vi "ReDraw ROI.vi"(6 "Mode (Redraw All)":T1, 8 "error in":errorcluster, 10 "Selected/Deselected":i32[](array[numeric]), 11 "XYZ Coordinates":T2[](array[typedef]) {"Apparent Frame Size" format="%#_6f"; "Original FOV (um)" format="%#_6f"; "Pixels per miniscan" format="%#_6f"; "Dwell Time per pixel" format="%#_6f"; "Resolution" format="%#_6f"; "ROI group ID" format="%#_6f"; "Laser Power (%)" format="%#_6f"; "Zoom" format="%#_6f"; "Frame Size" format="%#_6f"; "Number of lines" format="%#_6f"; "Composite ID" format="%#_6f"; "Angle (deg)" format="%#_6f"; "ROI Time (ns)" format="%#_6f"; "ROI ID" format="%#_6f"; "Pixels in ROI" format="%#_6f"; "ROI index" format="%#_6f"; "Z stop" format="%#_6f"; "Y stop" format="%#_6f"; "X stop" format="%#_6f"; "Z start" format="%#_6f"; "X start" format="%#_6f"; "Y start" format="%#_6f"}) -> (0 "error out":errorcluster)   [LabVIEW 2020]
uses:
  Visualisation/Functional Imaging Viewer/Typedefs/ROI parameters data type.ctl
  Typedefs/Redraw ROI.ctl
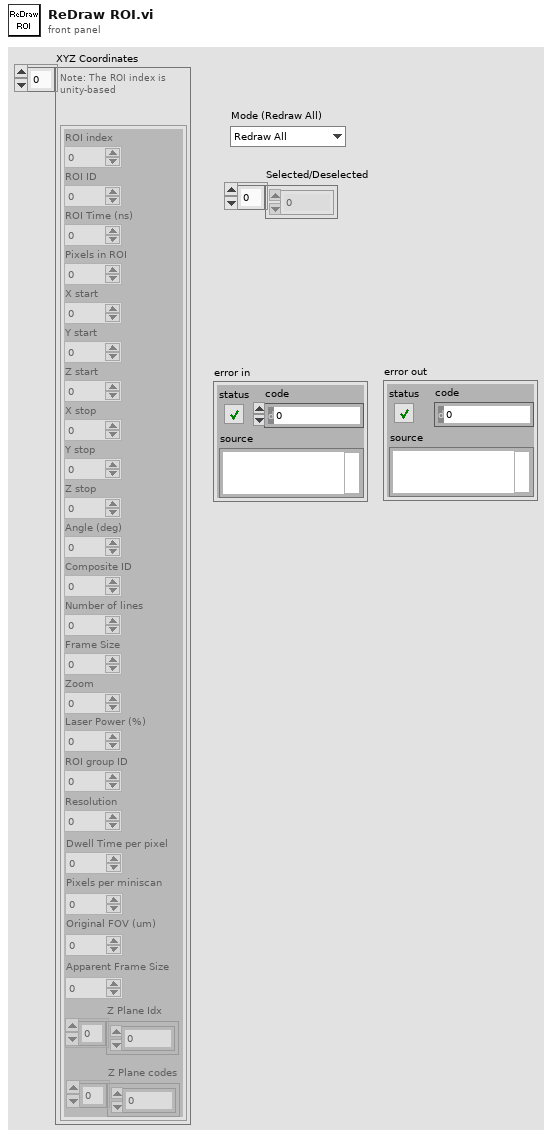
[diagram p1: front panel]
types:
  T1 = typedef "Redraw ROI.ctl" = enum16{"Redraw All", "Redraw Deselected", "Draw Last", "Redraw Selected"}
  T2 = typedef "ROI parameters data type.ctl" = cluster{"ROI index":dbl, "ROI ID":dbl, "ROI Time (ns)":dbl, "Pixels in ROI":dbl, "X start":dbl, "Y start":dbl, "Z start":dbl, "X stop":dbl, "Y stop":dbl, "Z stop":dbl, "Angle (deg)":dbl, "Composite ID":dbl, "Number of lines":dbl, "Frame Size":dbl, "Zoom":dbl, "Laser Power (%)":dbl, "ROI group ID":dbl, "Resolution":dbl, "Dwell Time per pixel":dbl, "Pixels per miniscan":dbl, "Original FOV (um)":dbl, "Apparent Frame Size":dbl, "Z Plane Idx":i32[], "Z Plane codes":i32[]}
  T3 = typedef "IMAQ Image.ctl" = refnum<image>
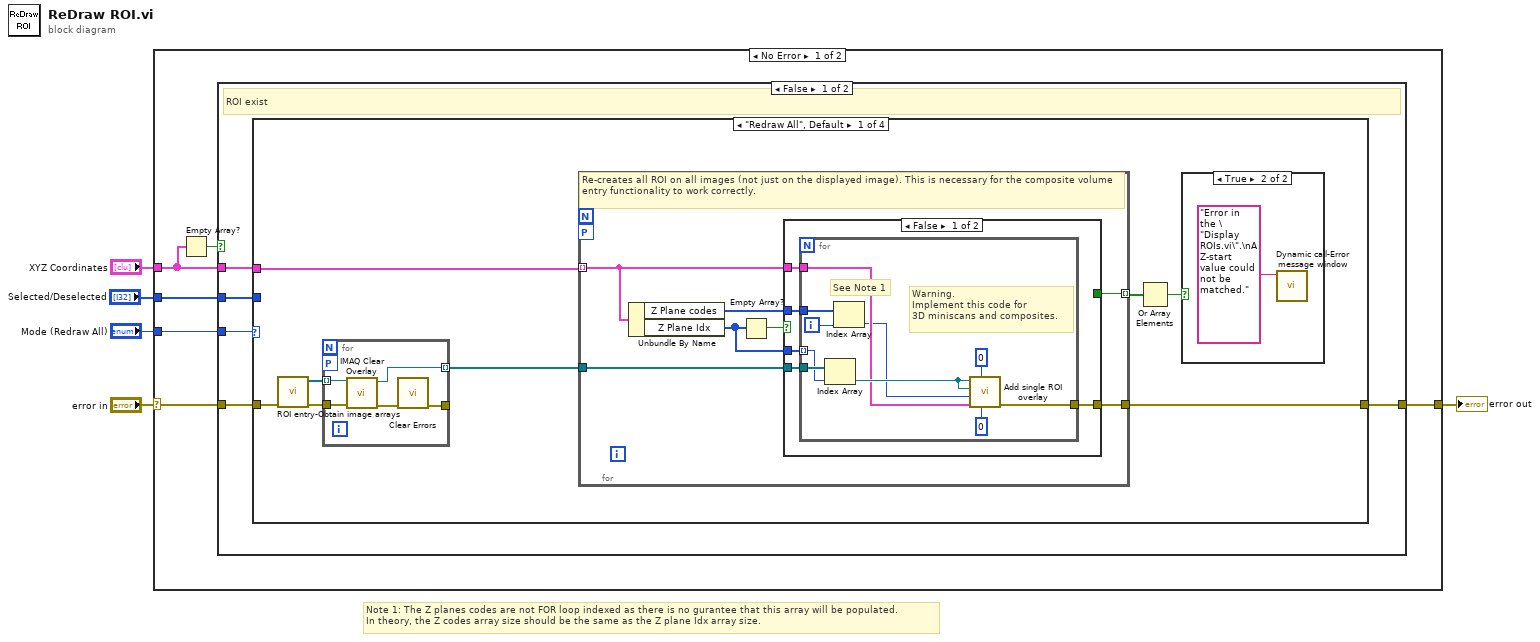
[diagram p0: block diagram]
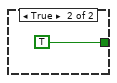
[diagram p3: hidden frame]
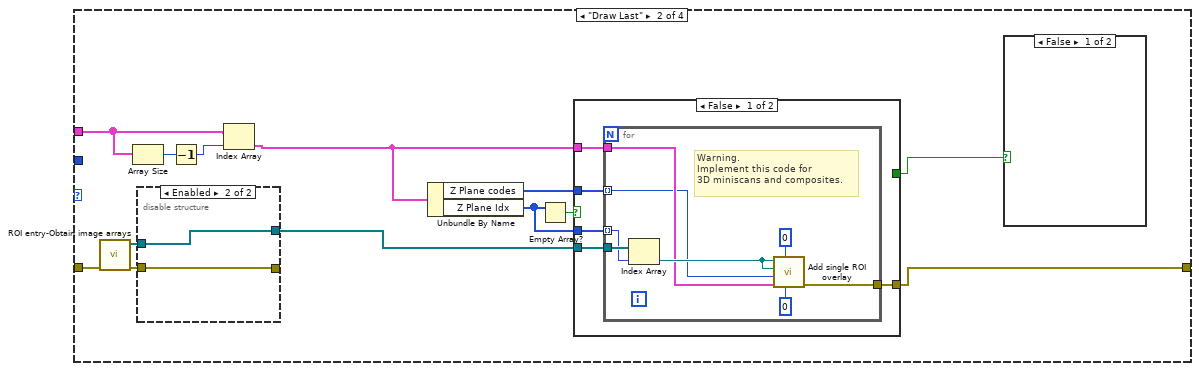
[diagram p4: hidden frame]
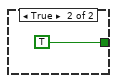
[diagram p5: hidden frame]
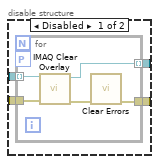
[diagram p6: hidden frame]
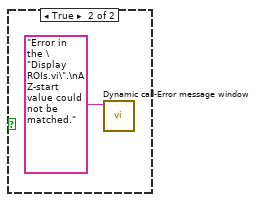
[diagram p7: hidden frame]
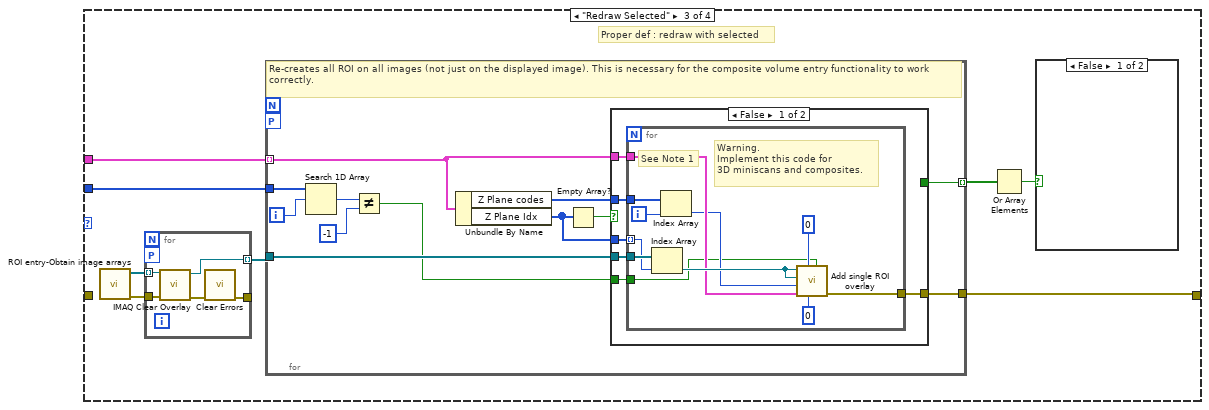
[diagram p8: hidden frame]
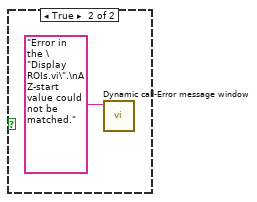
[diagram p9: hidden frame]
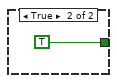
[diagram p10: hidden frame]
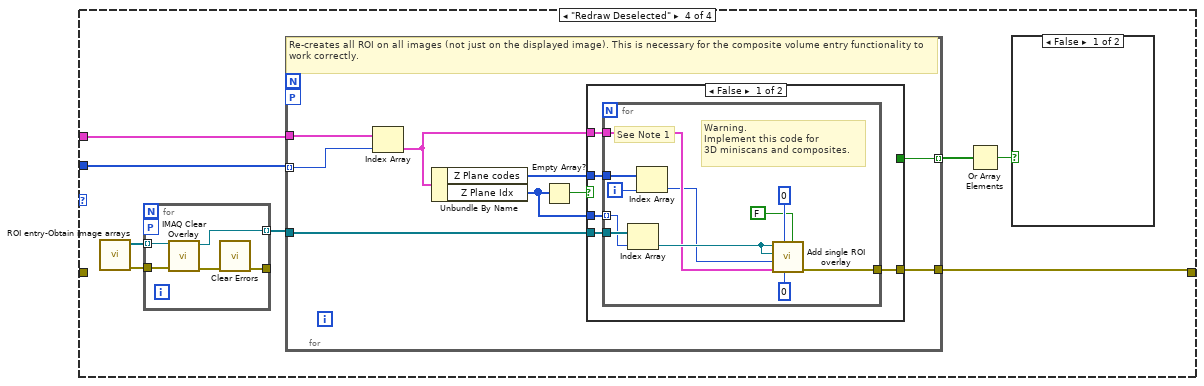
[diagram p11: hidden frame]
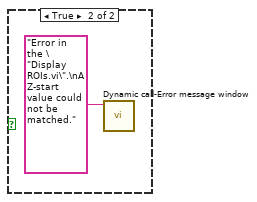
[diagram p12: hidden frame]
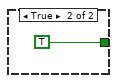
[diagram p13: hidden frame]
diagram:
  # "Note 1: The Z planes codes are not FOR loop indexed as there is no gurantee that this array will be populated.\nIn theory, the Z codes array size should be the same as the Z plane Idx array size."
  n1 = case shown="No Error" "error in" {
    selector: "error in" -> [w9 w178]
    tunnel: "XYZ Coordinates" -> [w11 _]
    tunnel: [w10 w178] -> w3
    tunnel: "Mode (Redraw All)" -> [w7 _]
    tunnel: "Selected/Deselected" -> [w6 _]
    frame No Error {
      n2 = Empty Array?(array=w11) -> (empty?=w8:bool)
      n3 = case shown="False" w8 {
        tunnel: w11 -> [w16 _]
        tunnel: [w15 w177] -> w10
        tunnel: w9 -> [w14 w177]
        tunnel: w7 -> [w13 _]
        tunnel: w6 -> [w12 _]
        frame False {
          # "ROI exist"
          n4 = case shown="\"Redraw All\", Default" w13 {
            tunnel: w16 -> [w24 w56 w94 w139]
            tunnel: [w20 w58 w95 w137] -> w15
            tunnel: w14 -> [w17 w64 _ _]
            tunnel: w12 -> [_ _ w93 w138]
            frame "Redraw All", Default {
              n5 = call "ROI entry-Obtain image arrays.vi"("error in (no error)"=w17) -> ("error IO"=w18:errorcluster, "RedImageArray"=w19:T3[])  [unwired: 9 in]
              n6 = for {
                tunnel: w19 -> [w30] mode=indexing
                tunnel: [w29] -> w23 mode=indexing
                workers-P: _ -> [_]
                tunnel: [w27] -> _
                tunnel: w18 -> [w26]
                n7 = call "IMAQ Clear Overlay"("error in (no error)"=w26, "Image"=w30) -> ("error out"=w28:errorcluster, "Image Out"=w29:T3)  [unwired: 8 in]
                n8 = call <vilib>:"Clear Errors.vi"("error in (no error)"=w28) -> ("error out"=w27:errorcluster)  [unwired: 5 in, 1 out]
              }
              n9 = for {
                tunnel: w24 -> [w33] mode=indexing
                tunnel: w23 -> [w37]
                workers-P: _ -> [_]
                tunnel: [w36] -> w22 mode=indexing
                tunnel: [w35] -> w20
                # "Re-creates all ROI on all images (not just on the displayed image). This is necessary for the composite volume entry functionality to work correctly."
                n10 = Unbundle By Name(w33) -> ("Z Plane codes"=w32:i32[], "Z Plane Idx"=w31:i32[])
                n11 = Empty Array?(array=w31) -> (empty?=w34:bool)
                n12 = case shown="False" w34 {
                  tunnel: w37 -> [w42 _]
                  tunnel: w33 -> [w41 _]
                  tunnel: [_ TRUE] -> w36
                  tunnel: [w40 _] -> w35
                  tunnel: w32 -> [w38 _]
                  tunnel: w31 -> [w39 _]
                  frame False {
                    n13 = for {
                      tunnel: w42 -> [w52]
                      tunnel: w41 -> [w50]
                      tunnel: [w47] -> w40
                      tunnel: w39 -> [w46] mode=indexing
                      tunnel: w38 -> [w45]
                      i -> [w44]
                      # "See Note 1"
                      # "Warning.\nImplement this code for\n3D miniscans and composites."
                      n14 = Index Array(array=w52, index=w46) -> (element=w51:T3)
                      n15 = Index Array(array=w45, index=w44) -> (element=w43:i32)
                      n16 = call "Add single ROI overlay.vi"("Abs. index of selected Z-plane (unity-based)"=0, "Number of Z-planes"=0, "ROI Properties"=w50, "Z code"=w43, "Image2"=w51, "Image1"=w51) -> ("Error out"=w47:errorcluster)  [unwired: 3 in, 2 out]
                    }
                  }
                  frame True {
                  }
                }
              }
              n17 = Or Array Elements(Boolean array=w22) -> (logical OR=w21:bool)
              n18 = case shown="True" w21 {
                frame False {
                }
                frame True {
                  n19 = call "Dynamic call-Error message window.vi"("Error Message"="Error in the \"Display ROIs.vi\".\nA Z-start value could not be matched.") -> ()  [unwired: 10 in, 1 out]
                }
              }
            }
            frame "Draw Last" {
              n20 = call "ROI entry-Obtain image arrays.vi"("error in (no error)"=w64) -> ("error IO"=w65:errorcluster, "RedImageArray"=w66:T3[])  [unwired: 9 in]
              n21 = Array Size(array=w56) -> (size(s)=w55:i32)
              n22 = disable-structure shown="Enabled" {
                disable-tunnel: [w84 w91] -> w60
                disable-tunnel: [w83 w90] -> _
                disable-tunnel: w66 -> [w82 w91]
                disable-tunnel: w65 -> [w81 w90]
                frame Disabled {
                  n23 = for {
                    tunnel: w82 -> [w89] mode=indexing
                    tunnel: [w88] -> w84 mode=indexing
                    workers-P: _ -> [_]
                    tunnel: [w86] -> w83
                    tunnel: w81 -> [w85]
                    n24 = call "IMAQ Clear Overlay"("error in (no error)"=w85, "Image"=w89) -> ("error out"=w87:errorcluster, "Image Out"=w88:T3)  [unwired: 8 in]
                    n25 = call <vilib>:"Clear Errors.vi"("error in (no error)"=w87) -> ("error out"=w86:errorcluster)  [unwired: 5 in, 1 out]
                  }
                }
                frame Enabled {
                }
              }
              n26 = Decrement(x=w55) -> (x-1=w54:i32)
              n27 = Index Array(array=w56, index=w54) -> (element=w57:T2)
              n28 = Unbundle By Name(w57) -> ("Z Plane codes"=w62:i32[], "Z Plane Idx"=w61:i32[])
              n29 = Empty Array?(array=w61) -> (empty?=w63:bool)
              n30 = case shown="False" w63 {
                tunnel: w60 -> [w71 _]
                tunnel: w57 -> [w70 _]
                tunnel: [_ TRUE] -> w59
                tunnel: [w69 _] -> w58
                tunnel: w62 -> [w67 _]
                tunnel: w61 -> [w68 _]
                frame False {
                  n31 = for {
                    tunnel: w71 -> [w79]
                    tunnel: w70 -> [w77]
                    tunnel: [w74] -> w69
                    tunnel: w68 -> [w73] mode=indexing
                    tunnel: w67 -> [w72] mode=indexing
                    # "Warning.\nImplement this code for\n3D miniscans and composites."
                    n32 = Index Array(array=w79, index=w73) -> (element=w78:T3)
                    n33 = call "Add single ROI overlay.vi"("Abs. index of selected Z-plane (unity-based)"=0, "Number of Z-planes"=0, "ROI Properties"=w77, "Z code"=w72, "Image2"=w78, "Image1"=w78) -> ("Error out"=w74:errorcluster)  [unwired: 3 in, 2 out]
                  }
                }
                frame True {
                }
              }
              n34 = case shown="False" w59 {
                frame False {
                }
                frame True {
                  n35 = call "Dynamic call-Error message window.vi"("Error Message"="Error in the \"Display ROIs.vi\".\nA Z-start value could not be matched.") -> ()  [unwired: 10 in, 1 out]
                }
              }
            }
            frame "Redraw Selected" {
              # "Proper def : redraw with selected"
              n36 = call "ROI entry-Obtain image arrays.vi"() -> ("error IO"=w99:errorcluster, "RedImageArray"=w100:T3[])  [unwired: 10 in]
              n37 = for {
                tunnel: w100 -> [w136] mode=indexing
                tunnel: [w135] -> w96 mode=indexing
                workers-P: _ -> [_]
                tunnel: [w133] -> _
                tunnel: w99 -> [w132]
                n38 = call "IMAQ Clear Overlay"("error in (no error)"=w132, "Image"=w136) -> ("error out"=w134:errorcluster, "Image Out"=w135:T3)  [unwired: 8 in]
                n39 = call <vilib>:"Clear Errors.vi"("error in (no error)"=w134) -> ("error out"=w133:errorcluster)  [unwired: 5 in, 1 out]
              }
              n40 = for {
                tunnel: w96 -> [w113]
                workers-P: _ -> [_]
                tunnel: [w112] -> w98 mode=indexing
                tunnel: [w111] -> w95
                tunnel: w94 -> [w107] mode=indexing
                tunnel: w93 -> [w106]
                i -> [w105]
                # "Re-creates all ROI on all images (not just on the displayed image). This is necessary for the composite volume entry functionality to work correctly."
                n41 = Search 1D Array(1D array=w106, element=w105) -> (index of element=w104:i32)  [unwired: 1 in]
                n42 = Not Equal?(x=w104, y=-1) -> (x != y?=w102:bool)
                n43 = Unbundle By Name(w107) -> ("Z Plane codes"=w109:i32[], "Z Plane Idx"=w108:i32[])
                n44 = Empty Array?(array=w108) -> (empty?=w110:bool)
                n45 = case shown="False" w110 {
                  tunnel: w113 -> [w119 _]
                  tunnel: w107 -> [w118 _]
                  tunnel: [_ TRUE] -> w112
                  tunnel: [w117 _] -> w111
                  tunnel: w109 -> [w115 _]
                  tunnel: w108 -> [w116 _]
                  tunnel: w102 -> [w114 _]
                  frame False {
                    n46 = for {
                      tunnel: w119 -> [w130]
                      tunnel: w118 -> [w128]
                      tunnel: [w125] -> w117
                      tunnel: w116 -> [w124] mode=indexing
                      tunnel: w115 -> [w123]
                      tunnel: w114 -> [w120]
                      i -> [w122]
                      # "See Note 1"
                      # "Warning.\nImplement this code for\n3D miniscans and composites."
                      n47 = Index Array(array=w130, index=w124) -> (element=w129:T3)
                      n48 = Index Array(array=w123, index=w122) -> (element=w121:i32)
                      n49 = call "Add single ROI overlay.vi"("Selected ?"=w120, "Abs. index of selected Z-plane (unity-based)"=0, "Number of Z-planes"=0, "ROI Properties"=w128, "Z code"=w121, "Image2"=w129, "Image1"=w129) -> ("Error out"=w125:errorcluster)  [unwired: 2 in, 2 out]
                    }
                  }
                  frame True {
                  }
                }
              }
              n50 = Or Array Elements(Boolean array=w98) -> (logical OR=w97:bool)
              n51 = case shown="False" w97 {
                frame False {
                }
                frame True {
                  n52 = call "Dynamic call-Error message window.vi"("Error Message"="Error in the \"Display ROIs.vi\".\nA Z-start value could not be matched.") -> ()  [unwired: 10 in, 1 out]
                }
              }
            }
            frame "Redraw Deselected" {
              n53 = call "ROI entry-Obtain image arrays.vi"() -> ("error IO"=w143:errorcluster, "RedImageArray"=w144:T3[])  [unwired: 10 in]
              n54 = for {
                tunnel: w144 -> [w176] mode=indexing
                tunnel: [w175] -> w140 mode=indexing
                workers-P: _ -> [_]
                tunnel: [w173] -> _
                tunnel: w143 -> [w172]
                n55 = call "IMAQ Clear Overlay"("error in (no error)"=w172, "Image"=w176) -> ("error out"=w174:errorcluster, "Image Out"=w175:T3)  [unwired: 8 in]
                n56 = call <vilib>:"Clear Errors.vi"("error in (no error)"=w174) -> ("error out"=w173:errorcluster)  [unwired: 5 in, 1 out]
              }
              n57 = for {
                tunnel: w140 -> [w154]
                workers-P: _ -> [_]
                tunnel: [w153] -> w142 mode=indexing
                tunnel: [w152] -> w137
                tunnel: w139 -> [w148]
                tunnel: w138 -> [w147] mode=indexing
                # "Re-creates all ROI on all images (not just on the displayed image). This is necessary for the composite volume entry functionality to work correctly."
                n58 = Index Array(array=w148, index=w147) -> (element=w146:T2)
                n59 = Unbundle By Name(w146) -> ("Z Plane codes"=w150:i32[], "Z Plane Idx"=w149:i32[])
                n60 = Empty Array?(array=w149) -> (empty?=w151:bool)
                n61 = case shown="False" w151 {
                  tunnel: w154 -> [w159 _]
                  tunnel: w146 -> [w158 _]
                  tunnel: [_ TRUE] -> w153
                  tunnel: [w157 _] -> w152
                  tunnel: w150 -> [w155 _]
                  tunnel: w149 -> [w156 _]
                  frame False {
                    n62 = for {
                      tunnel: w159 -> [w170]
                      tunnel: w158 -> [w168]
                      tunnel: [w165] -> w157
                      tunnel: w156 -> [w164] mode=indexing
                      tunnel: w155 -> [w163]
                      i -> [w162]
                      # "See Note 1"
                      # "Warning.\nImplement this code for\n3D miniscans and composites."
                      n63 = Index Array(array=w170, index=w164) -> (element=w169:T3)
                      n64 = Index Array(array=w163, index=w162) -> (element=w161:i32)
                      n65 = call "Add single ROI overlay.vi"("Selected ?"=FALSE, "Abs. index of selected Z-plane (unity-based)"=0, "Number of Z-planes"=0, "ROI Properties"=w168, "Z code"=w161, "Image2"=w169, "Image1"=w169) -> ("Error out"=w165:errorcluster)  [unwired: 2 in, 2 out]
                    }
                  }
                  frame True {
                  }
                }
              }
              n66 = Or Array Elements(Boolean array=w142) -> (logical OR=w141:bool)
              n67 = case shown="False" w141 {
                frame False {
                }
                frame True {
                  n68 = call "Dynamic call-Error message window.vi"("Error Message"="Error in the \"Display ROIs.vi\".\nA Z-start value could not be matched.") -> ()  [unwired: 10 in, 1 out]
                }
              }
            }
          }
        }
        frame True {
          # "ROI array is empty"
        }
      }
    }
    frame Error {
    }
  }
  "error out" <- w3
